vi "GraphSomething.vi"(1 "Graph This":dbl) -> (0 "Graph":cluster{dbl, "dt":dbl, dbl[]}(graph))   [LabVIEW 2013]
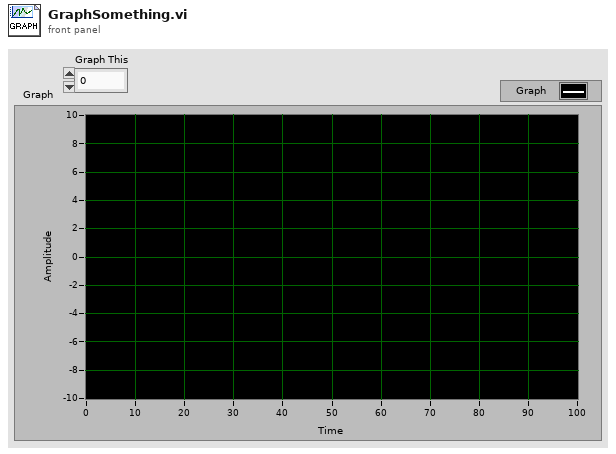
[diagram p1: front panel]
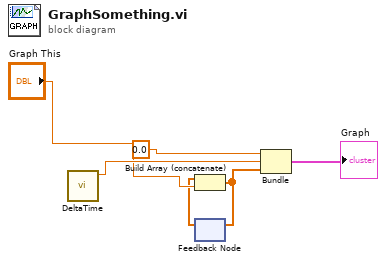
[diagram p0: block diagram]
diagram:
  n1 = call "DeltaTime.vi"() -> ("dt"=w6:dbl)  [unwired: 11 in]
  n2 = feedback #1() -> (w2:dbl[])  [unwired: 1 in]
  n3 = Build Array (concatenate)(w2, "Graph This") -> (w3:dbl[])
  n4 = feedback-in #1(w3) -> ()
  n5 = Bundle(0.0, "dt"=w6, w3) -> (→"Graph":cluster{dbl, "dt":dbl, dbl[]})  [unwired: 1 in]
